vi "TCP String Unbuilding.vi"(10 "data in":string, 11 "Array in":string[](array[string])) -> (3 "Array out":string[](array[string]))   [LabVIEW 2015]
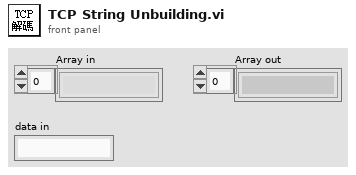
[diagram p1: front panel]
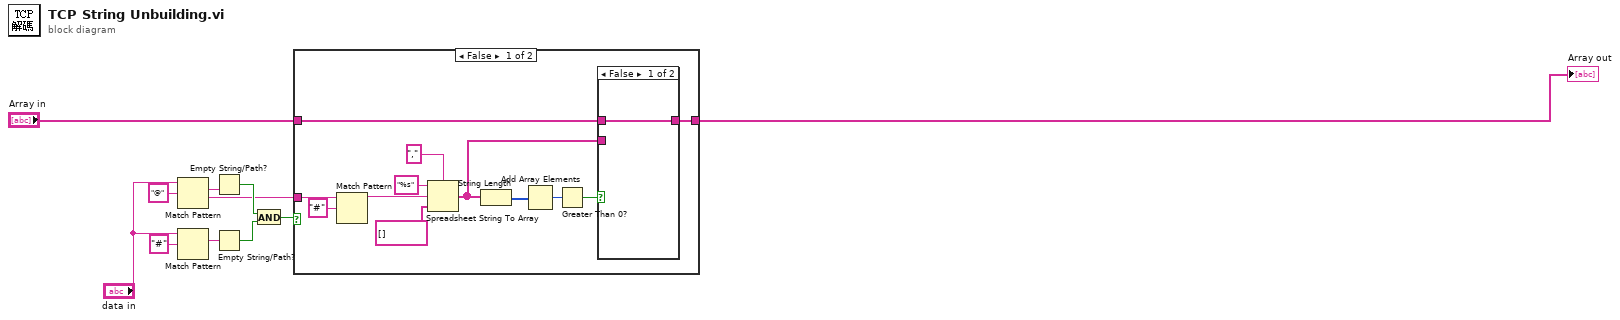
[diagram p0: block diagram]
diagram:
  n1 = Match Pattern(string="data in", regular expression="@") -> (match substring=w8:string, after substring=w4:string)  [unwired: 1 in, 2 out]
  n2 = Match Pattern(string="data in", regular expression="#") -> (match substring=w9:string)  [unwired: 1 in, 3 out]
  n3 = Empty String/Path?(string/path=w8) -> (empty?=w6:bool)
  n4 = Empty String/Path?(string/path=w9) -> (empty?=w7:bool)
  n5 = And(x=w6, y=w7) -> (x .and. y?=w5:bool)
  n6 = case shown="False" w5 {
    tunnel: "Array in" -> [w17 w26]
    tunnel: [w16 w26] -> w11
    tunnel: w4 -> [w14 _]
    frame False {
      n7 = Match Pattern(string=w14, regular expression="#") -> (before substring=w13:string)  [unwired: 1 in, 3 out]
      n8 = Spreadsheet String To Array(delimiter (Tab)=",", format string="%s", spreadsheet string=w13, array type (2D Dbl)=string[] []) -> (array=w18:string[])
      n9 = String Length(string=w18) -> (length=w22:i32[])
      n10 = Add Array Elements(numeric array=w22) -> (sum=w23:i32)
      n11 = Greater Than 0?(x=w23) -> (x > 0?=w12:bool)
      n12 = case shown="False" w12 {
        tunnel: w18 -> [_ w25]
        tunnel: [w24 w25] -> w16
        tunnel: w17 -> [w24 _]
        frame False {
        }
        frame True {
        }
      }
    }
    frame True {
    }
  }
  "Array out" <- w11
